vi "mongo_env_socket_connect.vi"(9 "port":i32, 10 "host":string, 11 "conn in":T1) -> (0 "error out":errorcluster, 3 "conn out":T1)   [LabVIEW 2013]
uses:
  mongo.ctl
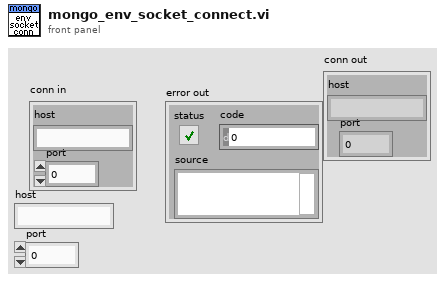
[diagram p1: front panel]
types:
  T1 = typedef "mongo.ctl" = cluster{"host":string, "port":i32}
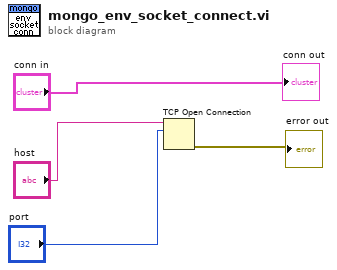
[diagram p0: block diagram]
diagram:
  n1 = TCP Open Connection(address="host", remote port or service name="port") -> (error out=→"error out":errorcluster)  [unwired: 3 in, 1 out]
  "conn out" <- "conn in"
